vi "_FPGA Turn LC Pump Off.vi"   [LabVIEW 2015]
uses:
  Type/_Syringe Pump Command.ctl
  Type/_RW Status.ctl
types:
  T1 = typedef "_Syringe Pump Command.ctl" = enum16{"start", "stop", "pause", "restart", "help", "set units", "set diameter", "set rate", "set time", "set volume", "set delay", "save setting", "read limit parameter", "view parameter", "status"}
  T2 = typedef "_RW Status.ctl" = enum8{"Done", "Do Read", "Do Write", "Set Latch1", "Set Latch2", "Set Latch3", "Set Latch4", "RP ON", "EL ON", "Serial Send", "Set LC Out", "Get LC In", "Read VAC", "Table Test", "Get Interlock", "Do Read2", "Do Write2"}
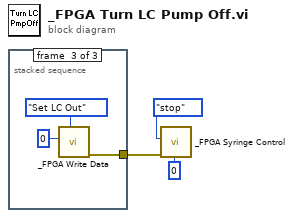
[diagram p0: block diagram]
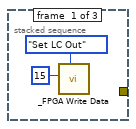
[diagram p2: hidden frame]
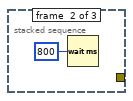
[diagram p3: hidden frame]
diagram:
  n1 = stacked-sequence {
    tunnel: [_ _ w7] -> w1
    frame #0 {
      n2 = call "_FPGA Write Data.vi"("Write Mode (Do Write)"=_RW_Status."Set LC Out", "Address"=u16 15) -> ()  [unwired: 4 in, 3 out]
    }
    frame #1 {
      n3 = Wait (ms)(milliseconds to wait=u32 800) -> ()  [unwired: 1 out]
    }
    frame #2 {
      n4 = call "_FPGA Write Data.vi"("Write Mode (Do Write)"=_RW_Status."Set LC Out", "Address"=u16 0) -> ("error out"=w7:errorcluster)  [unwired: 4 in, 2 out]
    }
  }
  n5 = call "_FPGA Syringe Control.vi"("Timeout (2s)"=u32 0, "error in (no error)"=w1, "Pump Command"=_Syringe_Pump_Command."stop") -> ()  [unwired: 3 in, 3 out]
